vi "FreqtoNote.vi"(0 "Freq meas":dbl) -> (1 "Note":string, 2 "Cents from note":dbl)   [LabVIEW 2015]
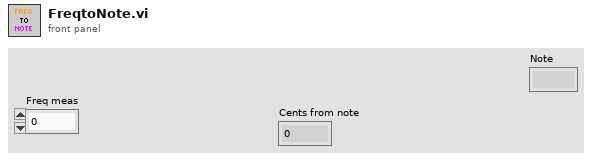
[diagram p1: front panel]
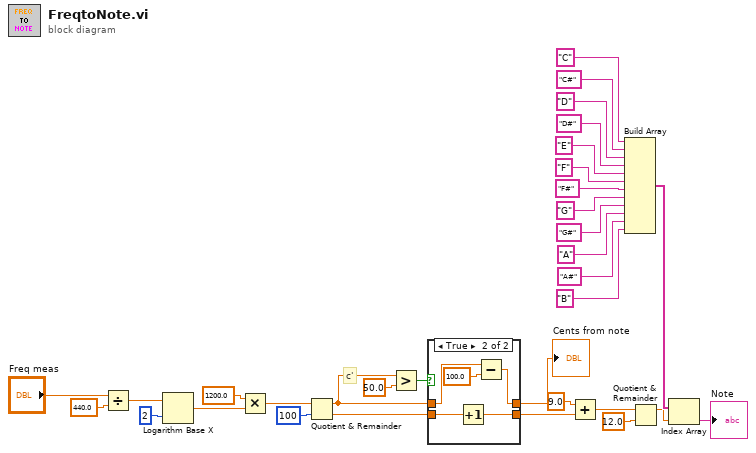
[diagram p0: block diagram]
diagram:
  # "c'"
  n1 = Divide(x="Freq meas", y=440.0 ("Freq const")) -> (x/y=w30:dbl)
  n2 = Logarithm Base X(1:2, 2:w30) -> (0:w13:dbl)
  n3 = Multiply(x=1200.0, y=w13) -> (x*y=w12:dbl)
  n4 = Quotient & Remainder(x=w12, y=100) -> (x-y*floor(x/y)=w9:dbl, floor(x/y)=w7:dbl)
  n5 = Greater?(x=w9, y=50.0 ("x")) -> (0:w11:bool)
  n6 = case shown="True" w11 {
    tunnel: w9 -> [w34 w38]
    tunnel: [w34 w37] -> w8
    tunnel: w7 -> [w33 w36]
    tunnel: [w33 w35] -> w2
    frame False {
    }
    frame True {
      n7 = Increment(x=w36) -> (x+1=w35:dbl)
      n8 = Subtract(x=w38, y=100.0) -> (x-y=w37:dbl)
    }
  }
  "Cents from note" <- w8
  n9 = Add(x=9.0, y=w2) -> (x+y=w6:dbl)
  n10 = Build Array("C", "C#", "D", "D#", "E", "F", "F#", "G", "G#", "A", "A#", "B") -> (w17:string[])
  n11 = Quotient & Remainder(x=w6, y=12.0) -> (x-y*floor(x/y)=w1:dbl)  [unwired: 1 out]
  n12 = Index Array(array=w17, index=w1) -> (element=→"Note":string)
